vi "Heartbeat reset.vi"(9 "New Beat":timestamp format="%<%x %.3X>T", 10 "Node ID":u8, 11 "CANopen in":refnum<class "CANopen.lvclass">) -> (3 "CANopen out":refnum<class "CANopen.lvclass">)   [LabVIEW 2026, in "canopen_.lvlib" / "CANopen.lvclass"]
doc: "Resets the watchdog of a specific heartbeat entry or of all the entries if \"Node ID\" is not specified. Resetting a watchdog means to put its \"Set value\" into its \"Value\"."
uses:
  CANopen.lvclass
  CANopen.lvclass/CANopen.ctl
  <vilib>/Utility/miscctls.llb/LVMapReplaceAction.ctl
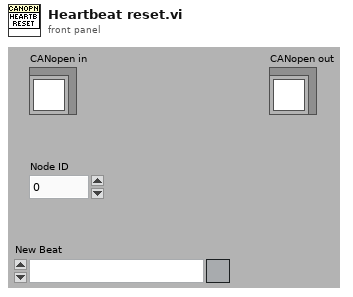
[diagram p1: front panel]
types:
  T1 = typedef "LVMapReplaceAction.ctl" = enum32{"Modify Entry only if found", "Add or Modify Entry", "Delete Entry"}
  T2 = map{u8, cluster{"Period":u16, "Timeout":u16, "Last Beat":timestamp}}
  T3 = cluster{"Period":u16, "Timeout":u16, "Last Beat":timestamp}
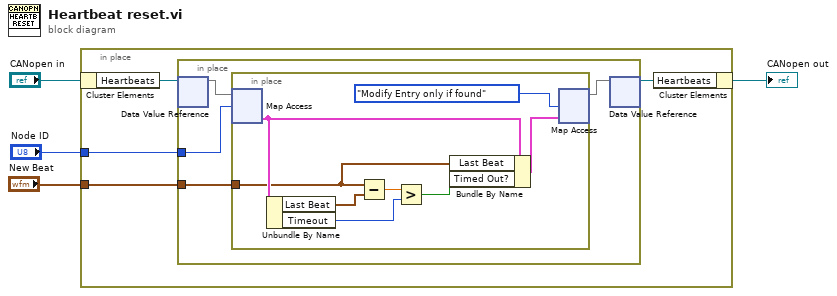
[diagram p0: block diagram]
diagram:
  n1 = in-place {
    in-place-border: "Node ID" -> [w8]
    in-place-border: "New Beat" -> [w7]
    n2 = in-place-cluster #1("CANopen in") -> ("Heartbeats"=w6:refnum<data-value>)
    n3 = in-place {
      in-place-border: w8 -> [w12]
      in-place-border: w7 -> [w11]
      n4 = in-place-dvr #2(w6) -> (w10:T2)  [unwired: 1 out]
      n5 = in-place {
        in-place-border: w11 -> [w14]
        n6 = in-place-map #3(w10, w12) -> (w18:T3)  [unwired: 1 in, 1 out]
        n7 = Unbundle By Name(w18) -> ("Last Beat"=w17:timestamp, "Timeout"=w15:u16)
        n8 = Subtract(x=w14, y=w17) -> (x-y=w16:dbl)
        n9 = Greater?(x=w16, y=w15) -> (0:w13:bool)
        n10 = Bundle By Name(cluster=w18, "Last Beat"=w14, "Timed Out?"=w13) -> (w20:T3)
        n11 = in-place-map #3(w20, LVMapReplaceAction."Modify Entry only if found" ("action")) -> (w9:T2)  [unwired: 2 out]
      }
      n12 = in-place-dvr #2(w9) -> (w5:refnum<data-value>)  [unwired: 1 out]
    }
    n13 = in-place-cluster #1("Heartbeats"=w5) -> (→"CANopen out":refnum<class "CANopen.lvclass">)
  }
